vi "UI Control and Indicator properties.vi"(7 "Enable Command":T1, 8 "Error In":errorcluster, 11 "Control Refnums":refnum<vi>[](array[refnum])) -> (0 "Error Out":errorcluster)   [LabVIEW 2012]
doc: "This SubVI carries out enable or disable of UI components passed to it as an 'array of control refnums'"
uses:
  UI Control and Indicator properties_Commands.ctl
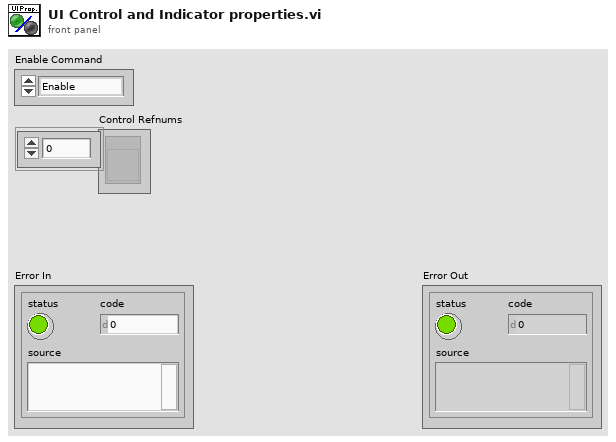
[diagram p1: front panel]
types:
  T1 = typedef "UI Control and Indicator properties_Commands.ctl" = enum16{"Enable", "Disable", "Disable and Grey", "Make Visible", "Make Invisible"}
  T2 = enum8{"Enabled", "Disabled", "Disabled and Grayed Out"}
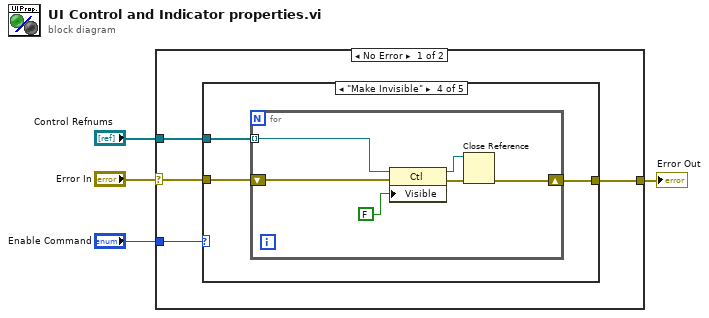
[diagram p0: block diagram]
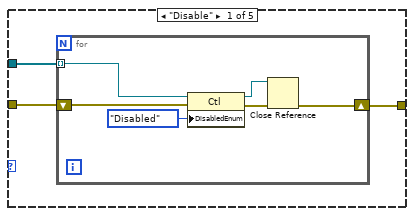
[diagram p2: hidden frame]
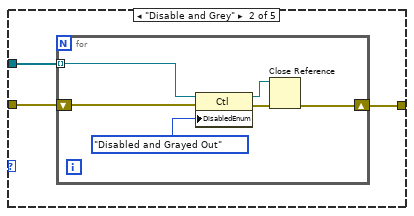
[diagram p3: hidden frame]
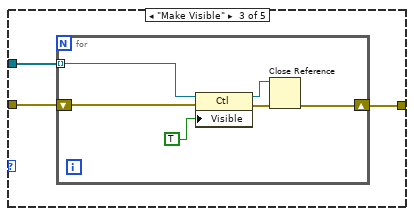
[diagram p4: hidden frame]
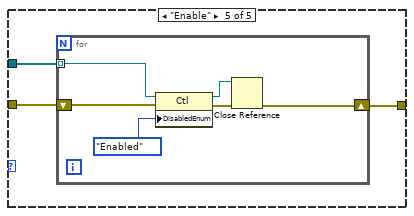
[diagram p5: hidden frame]
diagram:
  n1 = case shown="No Error" "Error In" {
    selector: "Error In" -> [w7 w54]
    tunnel: "Enable Command" -> [w8 _]
    tunnel: "Control Refnums" -> [w6 _]
    tunnel: [w5 w54] -> w1
    frame No Error {
      n2 = case shown="\"Make Invisible\"" w8 {
        tunnel: w7 -> [w10 w19 w28 w37 w46]
        tunnel: w6 -> [w11 w20 w29 w38 w47]
        tunnel: [w9 w18 w27 w36 w45] -> w5
        frame "Disable" {
          n3 = for {
            tunnel: w11 -> [w17] mode=indexing
            shift-right: [w14] -> w9
            shift-left: w10 -> [w16]
            n4 = property class="Ctl"(reference=w17, error in=w16, "DisabledEnum"=T2."Disabled" ("Disabled")) -> (reference out=w12:refnum<vi>, error out=w13:errorcluster)
            n5 = Close Reference(reference=w12, error in (no error)=w13) -> (error out=w14:errorcluster)
          }
        }
        frame "Disable and Grey" {
          n6 = for {
            tunnel: w20 -> [w26] mode=indexing
            shift-right: [w23] -> w18
            shift-left: w19 -> [w25]
            n7 = property class="Ctl"(reference=w26, error in=w25, "DisabledEnum"=T2."Disabled and Grayed Out" ("Disabled")) -> (reference out=w21:refnum<vi>, error out=w22:errorcluster)
            n8 = Close Reference(reference=w21, error in (no error)=w22) -> (error out=w23:errorcluster)
          }
        }
        frame "Make Visible" {
          n9 = for {
            tunnel: w29 -> [w35] mode=indexing
            shift-right: [w33] -> w27
            shift-left: w28 -> [w34]
            n10 = property class="Ctl"(reference=w35, error in=w34, "Visible"=TRUE) -> (reference out=w31:refnum<vi>, error out=w32:errorcluster)
            n11 = Close Reference(reference=w31, error in (no error)=w32) -> (error out=w33:errorcluster)
          }
        }
        frame "Make Invisible" {
          n12 = for {
            tunnel: w38 -> [w44] mode=indexing
            shift-right: [w42] -> w36
            shift-left: w37 -> [w43]
            n13 = property class="Ctl"(reference=w44, error in=w43, "Visible"=FALSE) -> (reference out=w40:refnum<vi>, error out=w41:errorcluster)
            n14 = Close Reference(reference=w40, error in (no error)=w41) -> (error out=w42:errorcluster)
          }
        }
        frame "Enable" {
          n15 = for {
            tunnel: w47 -> [w53] mode=indexing
            shift-right: [w48] -> w45
            shift-left: w46 -> [w52]
            n16 = property class="Ctl"(reference=w53, error in=w52, "DisabledEnum"=T2."Enabled" ("Disabled")) -> (reference out=w49:refnum<vi>, error out=w50:errorcluster)
            n17 = Close Reference(reference=w49, error in (no error)=w50) -> (error out=w48:errorcluster)
          }
        }
      }
    }
    frame Error {
    }
  }
  "Error Out" <- w1
